vi "Single_Measurement_sub_vi.vi"(0 "2182A VISA in":refnum<visa-resource-name>, 1 "2182A Error In":errorcluster, 2 "6221 VISA in":refnum<visa-resource-name>, 3 "6221 Error In":errorcluster, 4 "Current in (uA)":dbl, 6 "Start Time":u32, 7 "Meas. to Avg":i32, 8 "Outp. wait time (ms)":i32, 9 "Meas. wait time (ms)":i32) -> (5 "Current Change Registration Refnum":refnum<event-registration>, 13 "Measurement time":u32, 14 "2182A VISA out":refnum<visa-resource-name>, 15 "2182A Error Out":errorcluster, 16 "6221 VISA out":refnum<visa-resource-name>, 17 "6221 Error Out":errorcluster, 18 "Current out (uA)":dbl, 19 "Voltage (V)":dbl)   [LabVIEW 2014]
uses:
  <vilib>/Analysis/NI_AALBase.lvlib
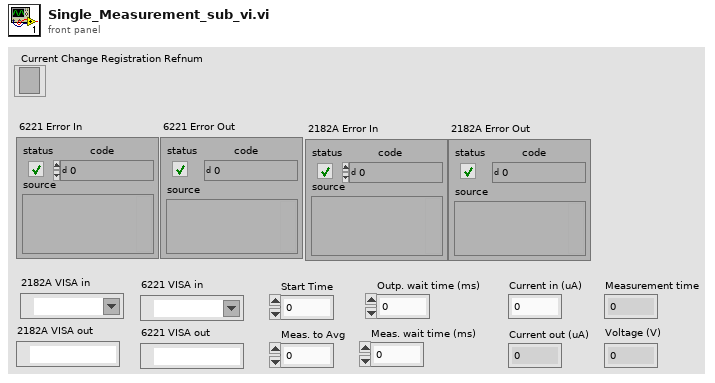
[diagram p1: front panel]
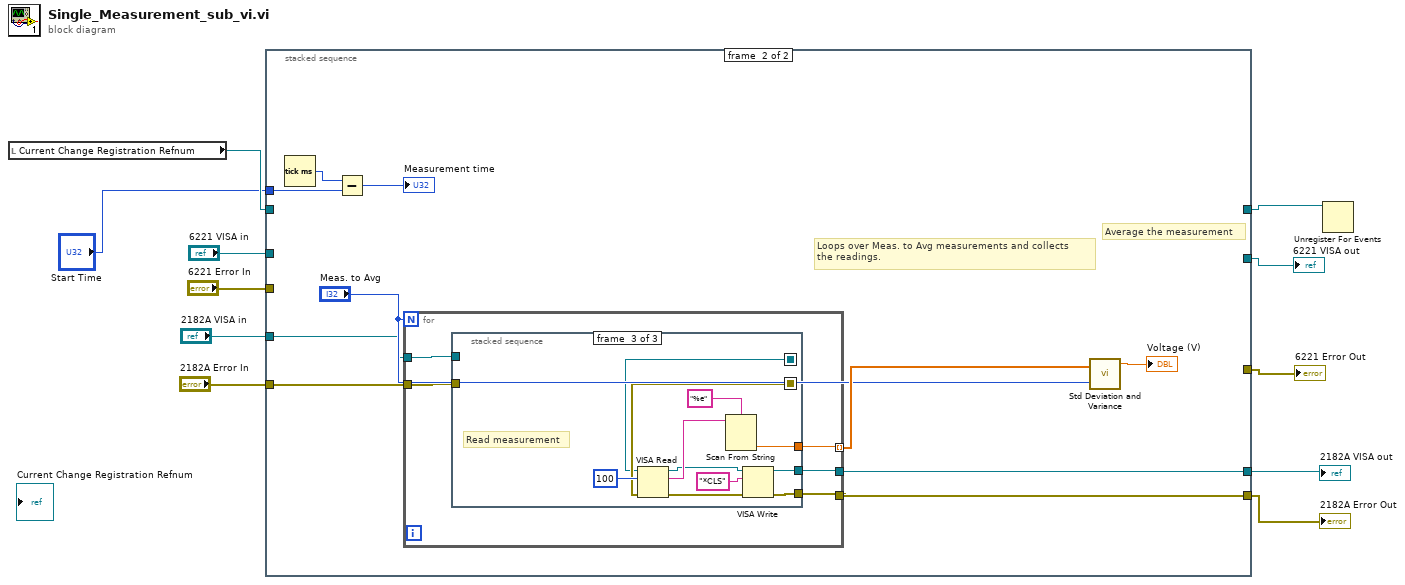
[diagram p0: block diagram]
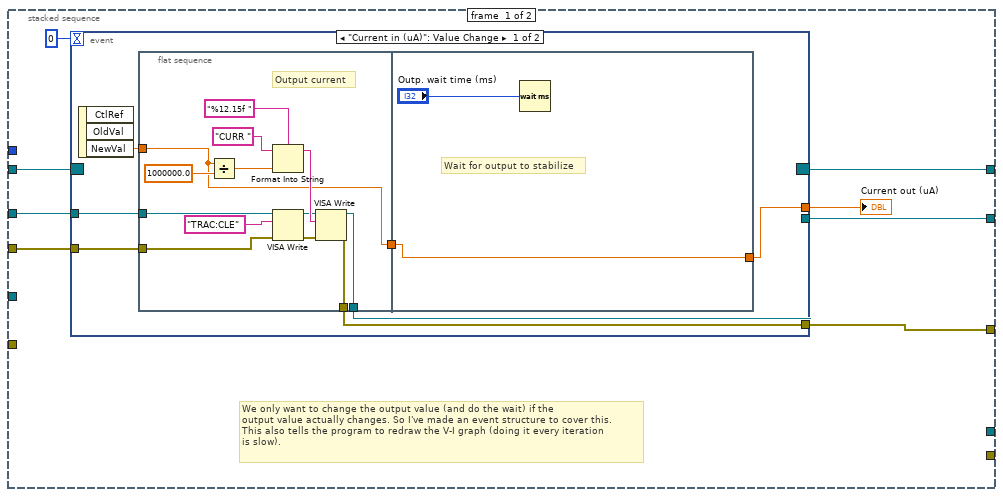
[diagram p2: hidden frame]
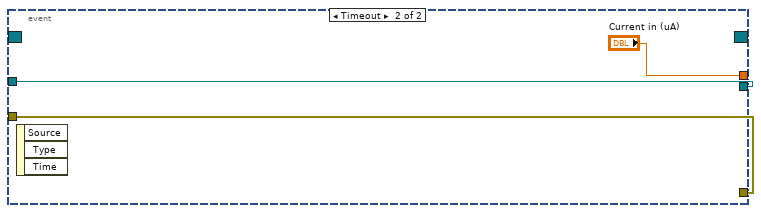
[diagram p3: hidden frame]
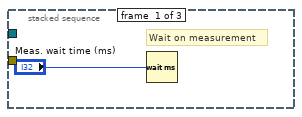
[diagram p4: hidden frame]
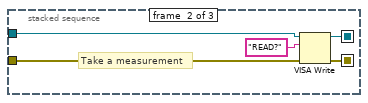
[diagram p5: hidden frame]
diagram:
  n1 = local read "Current Change Registration Refnum"() -> (w2:refnum<event-registration>)
  n2 = stacked-sequence {
    tunnel: "6221 Error In" -> [w18 _]
    tunnel: "2182A Error In" -> [_ w54]
    tunnel: "6221 VISA in" -> [w19 _]
    tunnel: "2182A VISA in" -> [_ w51]
    tunnel: w2 -> [w17 _]
    tunnel: "Start Time" -> [_ w49]
    tunnel: [w15 _] -> w7
    tunnel: [_ w46] -> w6
    tunnel: [_ w45] -> w5
    tunnel: [w13 _] -> w4
    tunnel: [w12 _] -> w3
    frame #0 {
      # "We only want to change the output value (and do the wait) if the\noutput value actually changes. So I've made an event structure to cover this.\nThis also tells the program to redraw the V-I graph (doing it every iteration\nis slow)."
      n3 = event shown="[0] \"Current in (uA)\": Value Change" {
        selector: w17 -> [_ _]
        dyn-events: [_ _] -> w15
        timeout: 0 -> [_ _]
        tunnel: w19 -> [w25 w42]
        tunnel: w18 -> [w24 w43]
        tunnel: [w22 "Current in (uA)"] -> w14
        tunnel: [w21 w42] -> w13
        tunnel: [w20 w43] -> w12
        event "Current in (uA)": Value Change {
          n4 = event-data() -> ("NewVal"=w26:dbl)  [unwired: 1 in, 2 out]
          n5 = flat-sequence {
            tunnel: w26 -> [w29]
            tunnel: w25 -> [w31]
            tunnel: w24 -> [w30]
            tunnel: [w29] -> w23
            tunnel: [w28] -> w21
            tunnel: [w27] -> w20
            tunnel: w23 -> [w40]
            tunnel: [w40] -> w22
            frame #0 {
              # "Output current"
              n6 = Divide(x=w29, y=1000000.0) -> (x/y=w34:dbl)
              n7 = Format Into String(format string="%12.15f ", initial string="CURR ", w34) -> (resulting string=w36:string)  [unwired: 1 in, 1 out]
              n8 = VISA Write(VISA resource name=w31, write buffer="TRAC:CLE", error in (no error)=w30) -> (VISA resource name out=w33:refnum<visa-resource-name>, error out=w38:errorcluster)  [unwired: 1 out]
              n9 = VISA Write(VISA resource name=w33, write buffer=w36, error in (no error)=w38) -> (VISA resource name out=w28:refnum<visa-resource-name>, error out=w27:errorcluster)  [unwired: 1 out]
            }
            frame #1 {
              # "Wait for output to stabilize"
              n10 = Wait (ms)(milliseconds to wait="Outp. wait time (ms)") -> ()  [unwired: 1 out]
            }
          }
        }
        event Timeout {
          n11 = event-data() -> ()  [unwired: 1 in, 3 out]
        }
      }
      "Current out (uA)" <- w14
    }
    frame #1 {
      # "Loops over Meas. to Avg measurements and collects\nthe readings."
      # "Average the measurement"
      n12 = Tick Count (ms)() -> (millisecond timer value=w50:u32)
      n13 = Subtract(x=w50, y=w49) -> (x-y=→"Measurement time":u32)
      n14 = for {
        N: "Meas. to Avg" -> [_]
        tunnel: w54 -> [w59]
        tunnel: [w58] -> w53 mode=indexing
        tunnel: w51 -> [w57]
        tunnel: [w56] -> w46
        tunnel: [w55] -> w45
        n15 = stacked-sequence {
          seq-local: [_ w63 _] -> [_ _ w75]
          seq-local: [_ w61 _] -> [_ _ w72]
          tunnel: w59 -> [_ w64 _]
          tunnel: [_ _ w73] -> w58
          tunnel: w57 -> [_ w62 _]
          tunnel: [_ _ w67] -> w56
          tunnel: [_ _ w66] -> w55
          frame #0 {
            # "Wait on measurement"
            n16 = Wait (ms)(milliseconds to wait="Meas. wait time (ms)") -> ()  [unwired: 1 out]
          }
          frame #1 {
            # "Take a measurement"
            n17 = VISA Write(VISA resource name=w62, write buffer="READ?", error in (no error)=w64) -> (VISA resource name out=w61:refnum<visa-resource-name>, error out=w63:errorcluster)  [unwired: 1 out]
          }
          frame #2 {
            # "Read measurement"
            n18 = VISA Read(VISA resource name=w72, byte count=100, error in (no error)=w75) -> (VISA resource name out=w69:refnum<visa-resource-name>, read buffer=w71:string, error out=w68:errorcluster)  [unwired: 1 out]
            n19 = Scan From String(format string="%e", input string=w71) -> (output 1=w73:dbl)  [unwired: 3 in, 3 out]
            n20 = VISA Write(VISA resource name=w69, write buffer="*CLS", error in (no error)=w68) -> (VISA resource name out=w67:refnum<visa-resource-name>, error out=w66:errorcluster)  [unwired: 1 out]
          }
        }
      }
      n21 = call <vilib>:"Std Deviation and Variance.vi"("X"=w53, "Weighting (Sample)"="Meas. to Avg") -> ("mean"=→"Voltage (V)":dbl)  [unwired: 2 out]
    }
  }
  "2182A Error Out" <- w5
  "6221 Error Out" <- w3
  "2182A VISA out" <- w6
  "6221 VISA out" <- w4
  n22 = Unregister For Events(event registration refnum=w7) -> ()  [unwired: 1 in, 1 out]
